vi "HDF5_array_mod.vi"(10 "delta":dbl, 11 "Array in":T1[][](array[typedef])) -> (3 "Array out":T1[][](array[typedef]))   [LabVIEW 2018]
doc: "Modify the incoming data to make it more interesting for test purposes.\nUpdate timestamps to current time."
uses:
  HDF5/HDF5_ToneInfoClust.ctl
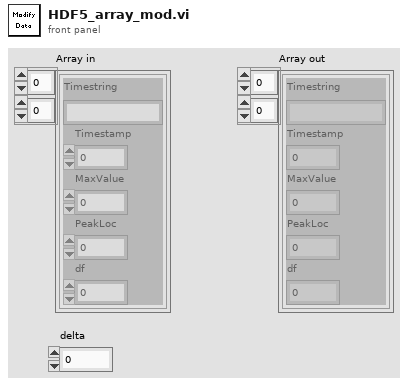
[diagram p1: front panel]
types:
  T1 = typedef "HDF5_ToneInfoClust.ctl" = cluster{"Timestring":string, "Timestamp":dbl, "MaxValue":dbl, "PeakLoc":dbl, "df":dbl}
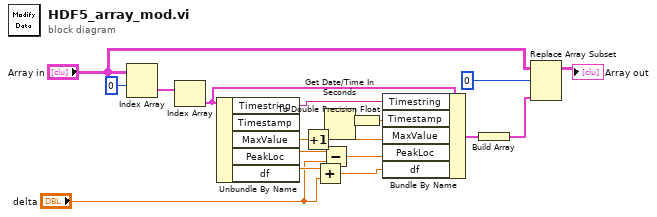
[diagram p0: block diagram]
diagram:
  n1 = Index Array(array="Array in", index (row)=0) -> (element=w17:T1[])  [unwired: 1 in]
  n2 = Index Array(array=w17) -> (element=w7:T1)  [unwired: 1 in]
  n3 = Unbundle By Name(w7) -> ("Timestring"=w8:string, "MaxValue"=w12:dbl, "PeakLoc"=w13:dbl, "df"=w14:dbl)  [unwired: 1 out]
  n4 = Increment(x=w12) -> (x+1=w10:dbl)
  n5 = Add(x=w14, y="delta") -> (x+y=w11:dbl)
  n6 = Subtract(x=w13, y="delta") -> (x-y=w9:dbl)
  n7 = Get Date/Time In Seconds() -> (seconds since 1Jan1904=w2:timestamp)
  n8 = To Double Precision Float(number=w2) -> (double precision float=w1:dbl)
  n9 = Bundle By Name(cluster=w7, "Timestring"=w8, "Timestamp"=w1, "MaxValue"=w10, "PeakLoc"=w9, "df"=w11) -> (w6:T1)
  n10 = Build Array(w6) -> (w4:T1[])
  n11 = Replace Array Subset(array="Array in", new element=w4, index (row)=0) -> (→"Array out":T1[][])  [unwired: 1 in]
